vi "Exit User Event.vi"(8 "error in (no error)":errorcluster) -> (0 "error out":errorcluster, 3 "Exit User Event":refnum<user-event>)   [LabVIEW 2018, in "Exit.lvlib"]
uses:
  Exit.lvlib
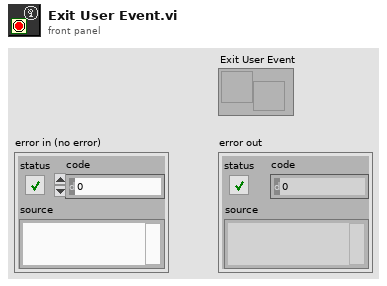
[diagram p1: front panel]
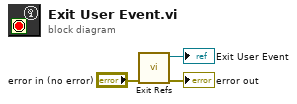
[diagram p0: block diagram]
diagram:
  n1 = call "Exit Refs.vi"("error in (no error)"="error in (no error)") -> ("error out"=→"error out":errorcluster, "Exit User Event"=→"Exit User Event":refnum<user-event>)  [unwired: 7 in, 2 out]
